vi "Create Channel Task.vi"(8 "error in (no error)":errorcluster, 10 "SQL query":string="SELECT max(MaximumVoltage),max(MinimumVoltage),max(SampleRate) FROM\nltt.daq_configuration \nWhere ChannelType='PWM_Input' and Enabled=1;", 11 "PWM Input in":refnum<class "PWM Input.lvclass">) -> (0 "error out":errorcluster, 3 "PWM Input out":refnum<class "PWM Input.lvclass">)   [LabVIEW 2023, in "HardwareAbstractionLayer_LVOOP.lvlib" / "PWM Input.lvclass"]
uses:
  PWM Input.lvclass
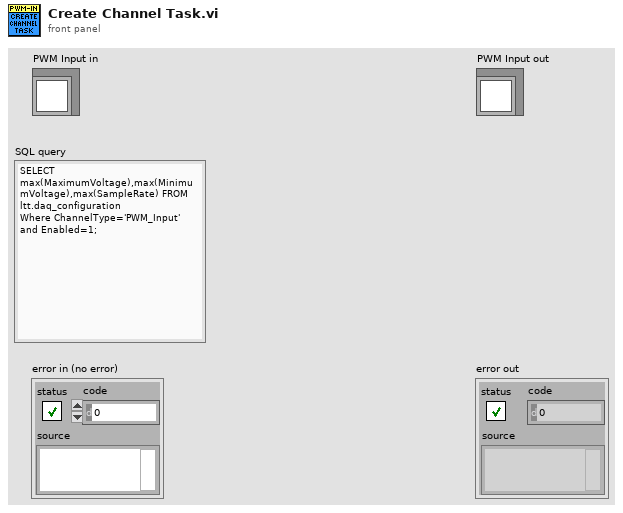
[diagram p1: front panel]
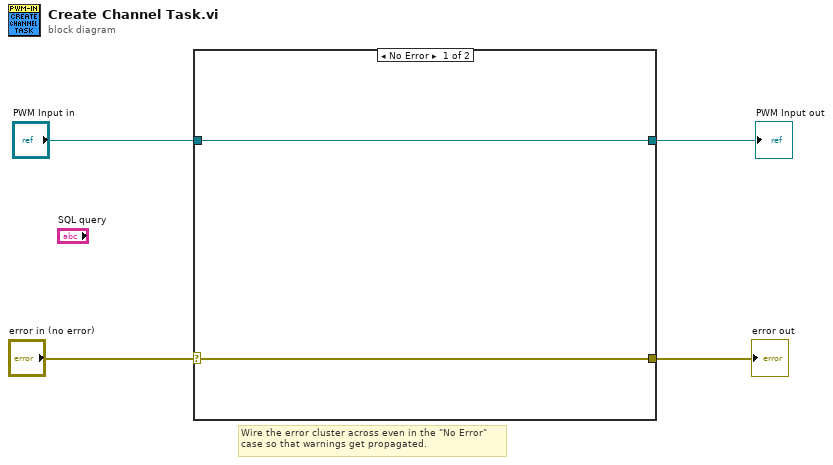
[diagram p0: block diagram]
diagram:
  # "Wire the error cluster across even in the \"No Error\"\ncase so that warnings get propagated."
  n1 = case shown="No Error" "error in (no error)" {
    selector: "error in (no error)" -> [w5 w8]
    tunnel: [w5 w8] -> w3
    tunnel: [w6 w7] -> w1
    tunnel: "PWM Input in" -> [w6 w7]
    frame No Error {
    }
    frame Error {
    }
  }
  "error out" <- w3
  "PWM Input out" <- w1
